vi "Generate Arguments.vi"(7 "subsystem?":bool, 8 "error in (no error)":errorcluster, 9 "command":string, 11 "client in":refnum<class "OpenSSH Client.lvclass">) -> (0 "error out":errorcluster, 2 "arguments":string[](array[string]), 3 "client out":refnum<class "OpenSSH Client.lvclass">, 5 "environment variables":cluster{"name":string, "value":string}[](array[cluster]))   [LabVIEW 2020, in "NI_SSH.lvlib" / "OpenSSH Client.lvclass"]
uses:
  <vilib>/net/SSH/Client/OpenSSH/OpenSSH Client.lvclass
  e:/builds/penguin/labview/branches/2020/dev/dist/vi.lib/net/SSH/Client/Generic/Generic Client.lvclass
  <vilib>/net/SSH/Client/Generic/Generic Client.lvclass/Generic Client.ctl
  <vilib>/net/SSH/Client/Generic/Read identity.vi
  <vilib>/net/SSH/Client/Generic/Read user_host.vi
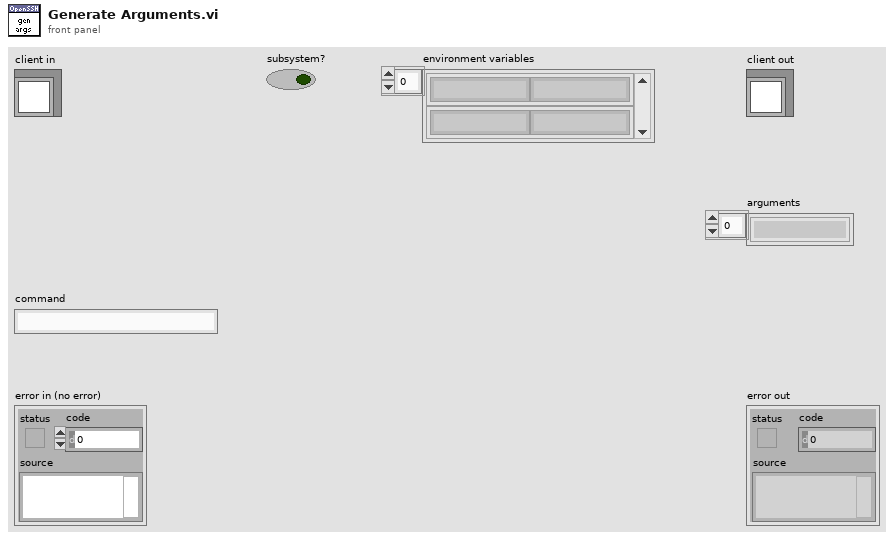
[diagram p1: front panel]
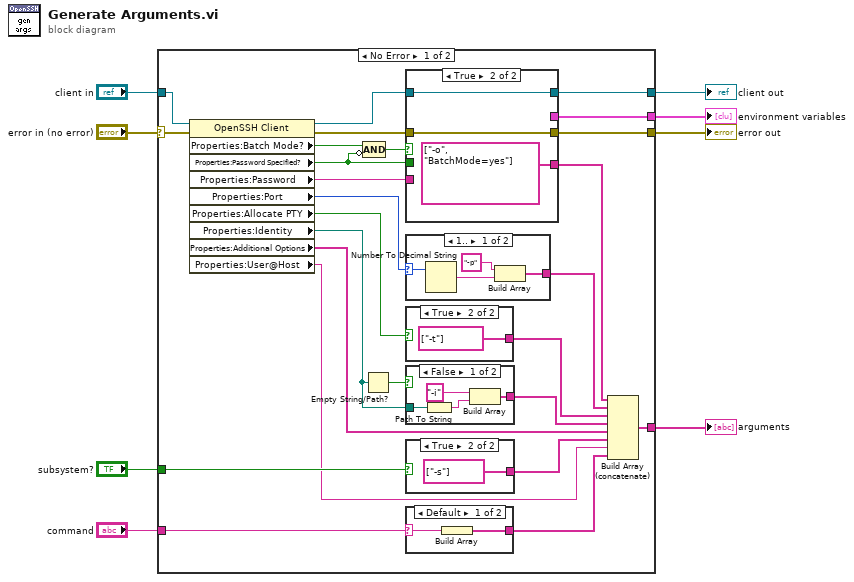
[diagram p0: block diagram]
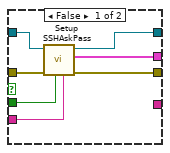
[diagram p6: hidden frame]
diagram:
  n1 = case shown="No Error" "error in (no error)" {
    selector: "error in (no error)" -> [w29 w57]
    tunnel: "client in" -> [w26 w58]
    tunnel: "subsystem?" -> [w33 _]
    tunnel: "command" -> [w31 _]
    tunnel: [w20 w58] -> w7
    tunnel: [w19 w57] -> w6
    tunnel: [w18 _] -> w5
    tunnel: [w17 _] -> w4
    frame No Error {
      n2 = property on="Property Node" class="OpenSSH Client"(reference=w26, error in=w29) -> (reference out=w27:refnum<class "OpenSSH Client.lvclass">, error out=w28:errorcluster, "Properties:Batch Mode?"=w16:bool, "Properties:Password Specified?"=w14:bool, "Properties:Password"=w13:string, "Properties:Port"=w30:u16, "Properties:Allocate PTY"=w22:bool, "Properties:Identity"=w11:path, "Properties:Additional Options"=w23:string[], "Properties:User@Host"=w9:string)
      n3 = Compound Arithmetic op=AND(w16, invert w14) -> (w15:bool)
      n4 = Empty String/Path?(string/path=w11) -> (empty?=w12:bool)
      n5 = case shown="True" w15 {
        tunnel: [w49 w51] -> w19
        tunnel: [w48 _] -> w18
        tunnel: [w47 w52] -> w20
        tunnel: w28 -> [w46 w51]
        tunnel: w27 -> [w45 w52]
        tunnel: [_ string[] ["-o", "BatchMode=yes"]] -> w24
        tunnel: w14 -> [w44 _]
        tunnel: w13 -> [w43 _]
        frame False {
          n6 = call <vilib>:"Setup SSHAskPass.vi"("password"=w43, "password specified?"=w44, "error in (no error)"=w46, "OpenSSH Client in"=w45) -> ("error out"=w49:errorcluster, "environment variables"=w48:cluster{"name":string, "value":string}[], "OpenSSH Client out"=w47:refnum<class "OpenSSH Client.lvclass">)  [unwired: 4 in, 1 out]
        }
        frame True {
        }
      }
      n7 = case shown="1.." w30 {
        selector: w30 -> [w54 _]
        tunnel: [w56 _] -> w34
        frame 1.. {
          n8 = Number To Decimal String(number=w54) -> (decimal integer string=w53:string)  [unwired: 1 in]
          n9 = Build Array("-p", w53) -> (w56:string[])
        }
        frame ..0 {
        }
      }
      n10 = case shown="True" w22 {
        tunnel: [_ string[] ["-t"]] -> w21
        frame False {
        }
        frame True {
        }
      }
      n11 = case shown="False" w12 {
        tunnel: w11 -> [w39 _]
        tunnel: [w38 _] -> w10
        frame False {
          n12 = Path To String(path=w39) -> (string=w40:string)
          n13 = Build Array("-i", w40) -> (w38:string[])
        }
        frame True {
        }
      }
      n14 = case shown="True" w33 {
        tunnel: [_ string[] ["-s"]] -> w25
        frame False {
        }
        frame True {
        }
      }
      n15 = case shown="Default" w31 {
        selector: w31 -> [w37 _]
        tunnel: [w36 _] -> w32
        frame Default {
          n16 = Build Array(w37) -> (w36:string[])
        }
        frame "" {
        }
      }
      n17 = Build Array (concatenate)(w24, w34, w21, w10, w23, w25, w9, w32) -> (w17:string[])
    }
    frame Error {
    }
  }
  "error out" <- w6
  "client out" <- w7
  "arguments" <- w4
  "environment variables" <- w5
